vi "User Console - Fire Transaction.vi"(8 "error in (no error)":errorcluster, 10 "Transaction":T1, 11 "View Model":T2) -> (0 "error out":errorcluster, 3 "View Model":T2)   [LabVIEW 2017]
doc: "Generate user Event for selected Transaction."
uses:
  View Model/Controls/View Model.ctl
  View Model/Controls/Shared Model.ctl
  Error Handler/Controls/Error Model.ctl
  Error Handler/Controls/Error Data.ctl
  Error Handler/Controls/Error Type.ctl
  Error Handler/Controls/Error Source.ctl
  Configuration/Controls/Config Model.ctl
  Configuration/Controls/Config CMD.ctl
  Configuration/Controls/Config Command.ctl
  Controller/Controls/Controller Model.ctl
  Controller/Controls/Controller Overhead.ctl
  Controller/Controls/Controller Transaction.ctl
  Controller/Controls/Controller State.ctl
  Configuration/Controls/Config Data Record.ctl
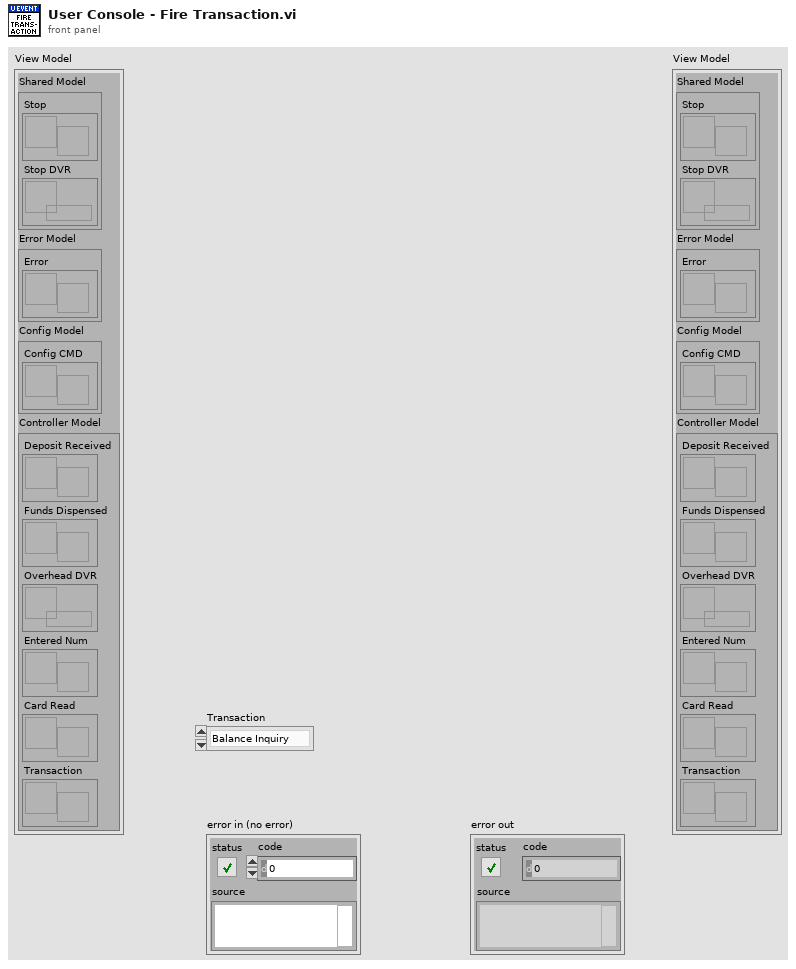
[diagram p1: front panel]
types:
  T1 = typedef "Controller Transaction.ctl" = enum16{"Balance Inquiry", "Deposit", "Withdrawal", "Fast Cash", "New Transaction", "Terminate Session"}
  T2 = typedef "View Model.ctl" = cluster{"Shared Model":T3, "Error Model":T4, "Config Model":T5, "Controller Model":T6}
  T3 = typedef "Shared Model.ctl" = cluster{"Stop":refnum<user-event>, "Stop DVR":refnum<data-value>}
  T4 = typedef "Error Model.ctl" = cluster{"Error":refnum<user-event>}
  T5 = typedef "Config Model.ctl" = cluster{"Config CMD":refnum<user-event>}
  T6 = typedef "Controller Model.ctl" = cluster{"Deposit Received":refnum<user-event>, "Funds Dispensed":refnum<user-event>, "Overhead DVR":refnum<data-value>, "Entered Num":refnum<user-event>, "Card Read":refnum<user-event>, "Transaction":refnum<user-event>}
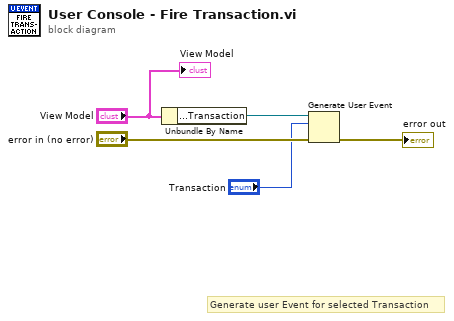
[diagram p0: block diagram]
diagram:
  # "Generate user Event for selected Transaction"
  n1 = Unbundle By Name("View Model") -> ("Controller Model.Transaction"=w5:refnum<user-event>)
  n2 = Generate User Event(user event=w5, event data cluster="Transaction", error in="error in (no error)") -> (error out=→"error out":errorcluster)  [unwired: 1 in, 1 out]
  "View Model" <- "View Model"
